vi "Add Attribute - Datetime.vi"(8 "error in (no error)":errorcluster, 9 "Value":timestamp caption="Value (00:00:00.000 DD/MM/YYYY)", 10 "Attribute":string, 11 "YAML Parser in":refnum<class "YAML Parser.lvclass">) -> (0 "error out":errorcluster, 3 "YAML Parser out":refnum<class "YAML Parser.lvclass">)   [LabVIEW 2015, in "YAML Parser.lvclass"]
uses:
  YAML Parser.lvclass
  YAML Parser.lvclass/YAML Parser.ctl
panel:
  out "replaced":bool
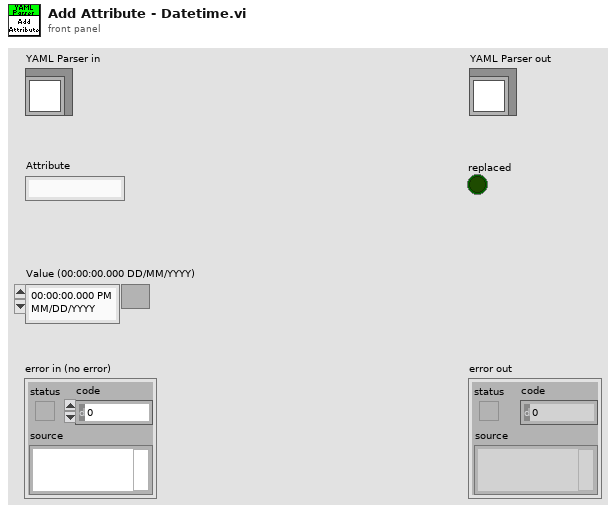
[diagram p1: front panel]
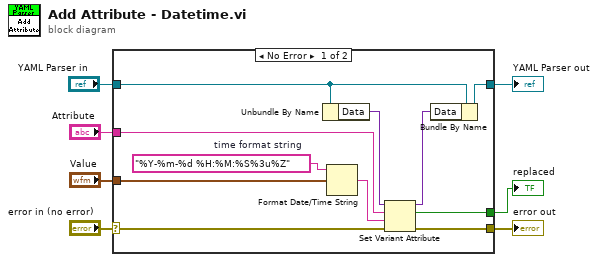
[diagram p0: block diagram]
diagram:
  n1 = case shown="No Error" "error in (no error)" {
    selector: "error in (no error)" -> [w16 w20]
    tunnel: [w15 w20] -> w6
    tunnel: [w18 w19] -> w4
    tunnel: "YAML Parser in" -> [w17 w19]
    tunnel: "Attribute" -> [w12 _]
    tunnel: "Value" -> [w11 _]
    tunnel: [w10 _] -> w1
    frame No Error {
      w8 = "%Y-%m-%d %H:%M:%S%3u%Z"  # time format string
      n2 = Unbundle By Name(w17) -> ("Data"=w14:variant)
      n3 = Format Date/Time String(time format string (%c)=w8, seconds (now)=w11) -> (date/time string=w9:string)  [unwired: 1 in]
      n4 = Set Variant Attribute(Variant=w14, name=w12, value=w9, error in=w16) -> (Variant out=w13:variant, replaced=w10:bool, error out=w15:errorcluster)
      n5 = Bundle By Name(cluster=w17, "Data"=w13) -> (w18:refnum<class "YAML Parser.lvclass">)
    }
    frame Error {
    }
  }
  "error out" <- w6
  "YAML Parser out" <- w4
  "replaced" <- w1
